vi "Ramp.vi"(7 "Points":i32, 9 "End Angle":dbl, 10 "Start Angle":dbl, 11 "Array In":dbl[](array[numeric])) -> (2 "Last Value":dbl, 3 "Array Out":dbl[](array[numeric]))   [LabVIEW 2018]
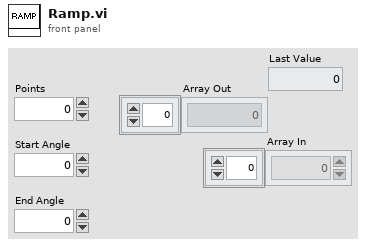
[diagram p1: front panel]
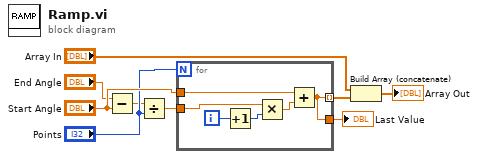
[diagram p0: block diagram]
diagram:
  n1 = Subtract(x="End Angle", y="Start Angle") -> (x-y=w6:dbl)
  n2 = Divide(x=w6, y="Points") -> (x/y=w8:dbl)
  n3 = for {
    N: "Points" -> [_]
    tunnel: w8 -> [w15]
    tunnel: [w10] -> w3 mode=indexing
    tunnel: "Start Angle" -> [w11]
    tunnel: [w10] -> w1
    i -> [w14]
    n4 = Increment(x=w14) -> (x+1=w12:i32)
    n5 = Multiply(x=w15, y=w12) -> (x*y=w13:dbl)
    n6 = Add(x=w11, y=w13) -> (x+y=w10:dbl)
  }
  "Last Value" <- w1
  n7 = Build Array (concatenate)("Array In", w3) -> (→"Array Out":dbl[])
